vi "GetFirstDeviceKey.vi"(8 "error in (no error)":errorcluster, 11 "USBLib In":refnum<k24>) -> (0 "error out":errorcluster, 1 "Device Key":string, 3 "USBLib Out":refnum<k24>)   [LabVIEW 2009]
uses:
  C:/Samples/LabVIEW/UseDeviceKey/LabVIEW 2009/UseDeviceKey (with Device VIs)/UsbDllWrap.dll
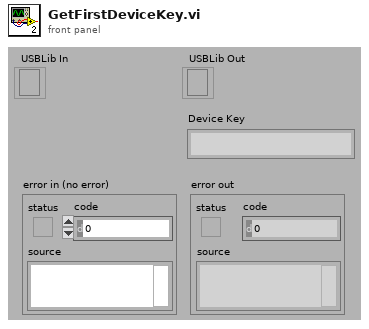
[diagram p1: front panel]
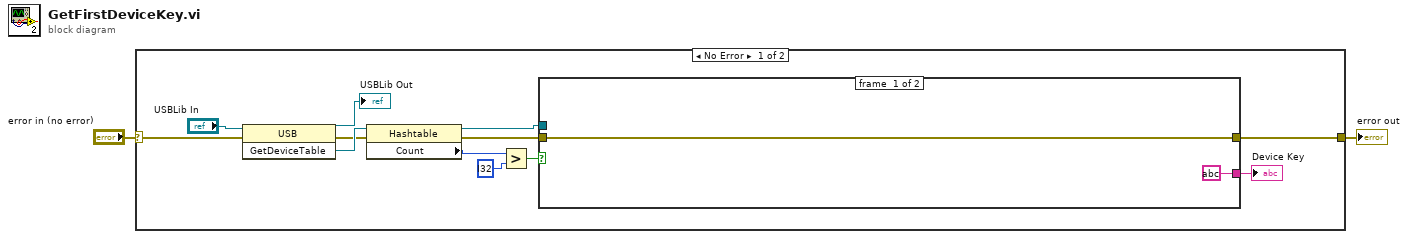
[diagram p0: block diagram]
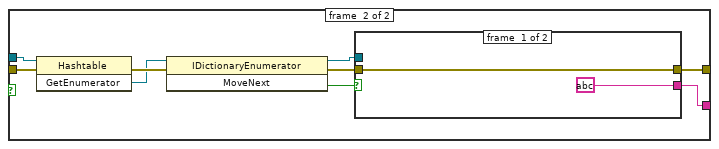
[diagram p2: hidden frame]
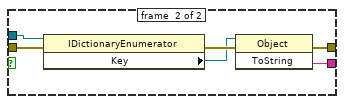
[diagram p3: hidden frame]
diagram:
  n1 = case shown="No Error" "error in (no error)" {
    selector: "error in (no error)" -> [w5 w34]
    tunnel: [w8 w34] -> w2
    frame #0 {
      n2 = invoke class="USB" method="GetDeviceTable"(reference="USBLib In", error in=w5) -> (reference out=→"USBLib Out":refnum<k24>, error out=w4:errorcluster, "GetDeviceTable"=w7:refnum<k24>)  [unwired: 1 in]
      n3 = property class="Hashtable"(reference=w7, error in=w4) -> (reference out=w10:refnum<k24>, error out=w9:errorcluster, "Count"=w14:i32)
      n4 = Greater?(x=w14, y=i32 ?) -> (0:w12:bool)
      n5 = case shown="True" w12 {
        tunnel: [string ? w20] -> w11
        tunnel: w10 -> [_ w25]
        tunnel: w9 -> [w15 w24]
        tunnel: [w15 w17] -> w8
        frame #0 {
        }
        frame #1 {
          n6 = invoke class="Hashtable" method="GetEnumerator"(reference=w25, error in=w24) -> (error out=w23:errorcluster, "GetEnumerator"=w22:refnum<k24>)  [unwired: 1 in, 1 out]
          n7 = invoke class="IDictionaryEnumerator" method="MoveNext"(reference=w22, error in=w23) -> (reference out=w19:refnum<k24>, error out=w18:errorcluster, "MoveNext"=w21:bool)  [unwired: 1 in]
          n8 = case shown="True" w21 {
            tunnel: [string ? w31] -> w20
            tunnel: w19 -> [_ w33]
            tunnel: w18 -> [w26 w32]
            tunnel: [w26 w30] -> w17
            frame #0 {
            }
            frame #1 {
              n9 = property class="IDictionaryEnumerator"(reference=w33, error in=w32) -> (error out=w29:errorcluster, "Key"=w28:refnum<k24>)  [unwired: 1 out]
              n10 = invoke class="Object" method="ToString"(reference=w28, error in=w29) -> (error out=w30:errorcluster, "ToString"=w31:string)  [unwired: 1 in, 1 out]
            }
          }
        }
      }
      "Device Key" <- w11
    }
    frame #1 {
    }
  }
  "error out" <- w2
